vi "ExDisplayMultiple.vi"() -> ()   [LabVIEW 2010]
uses:
  GlobalCurrentFrame.vi
  GlobalFileInfo.vi
  GlobalLastFrame.vi
panel:
  out "Last Frame Number":u32
  in  "Stop 2":bool
  in  "Stop":bool
  out "Current Frame Number":u32
  in  "Go To End":bool
  in  "Go to begining":bool
  in  "Prev Frame":bool
  in  "Next Frame":bool
  in  "Full File Name":path
  out "error out":errorcluster
  in  "error in (no error)":errorcluster
  in  "SITKFULLDISPLAYLib.SITKFullDisplay":refnum<k7>(container)
  # "Browse match pattern is set to *.tif.  Modify this if different file type is needed."
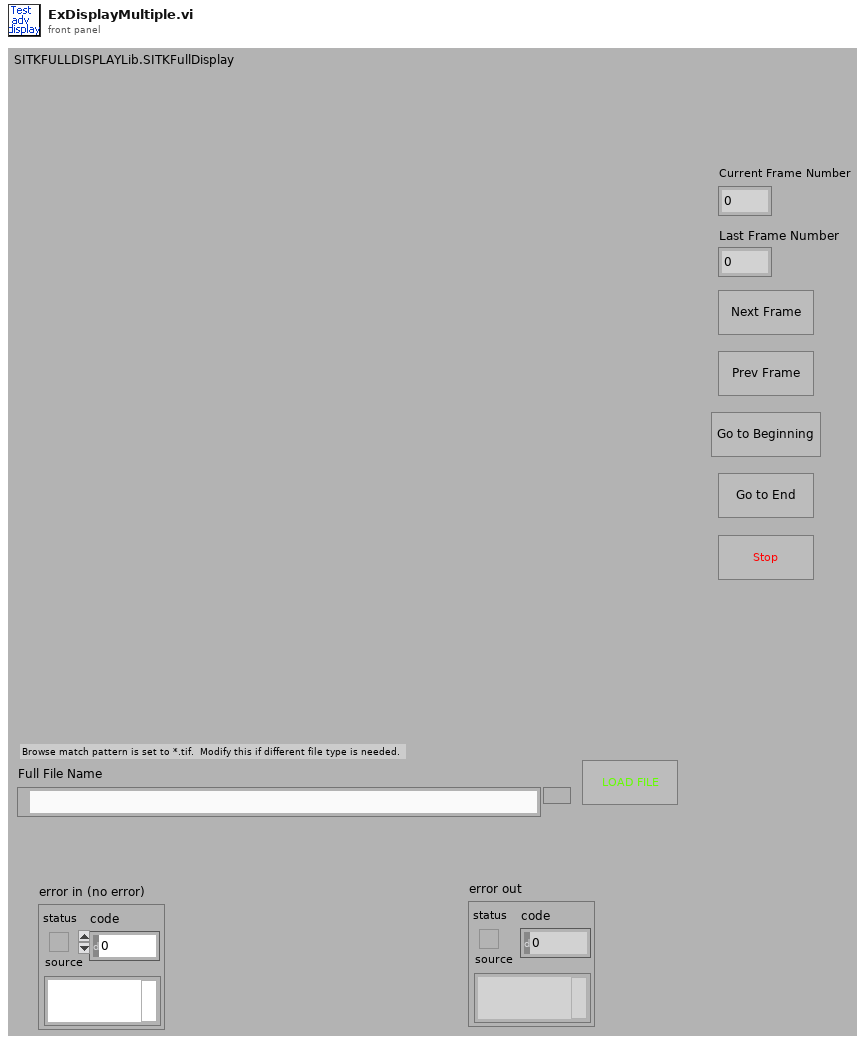
[diagram p1: front panel]
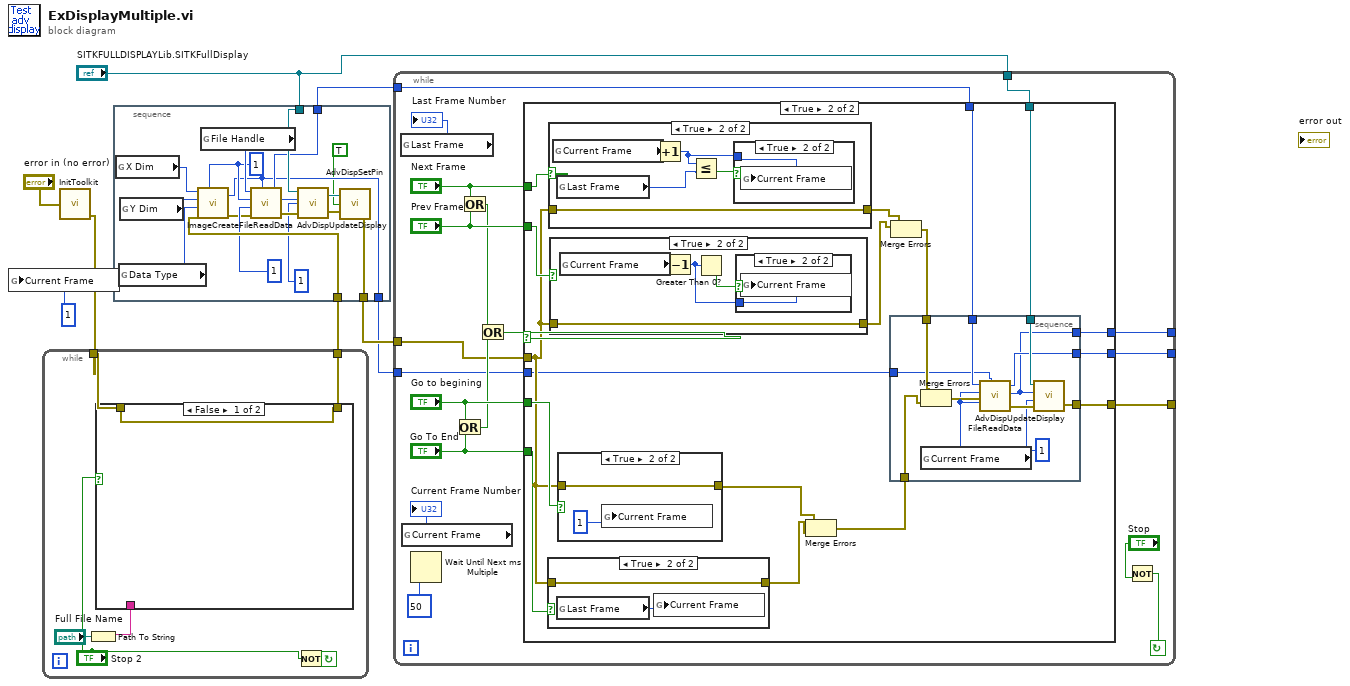
[diagram p0: block diagram]
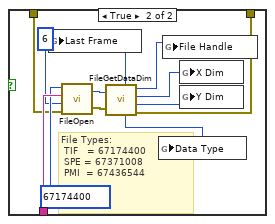
[diagram p2: hidden frame]
diagram:
  n1 = global write "GlobalCurrentFrame.vi" "Current Frame"(1) -> ()
  n2 = call <userlib>:"InitToolkit.vi"("error in"="error in (no error)") -> ("error out"=w4:errorcluster)
  n3 = while {
    tunnel: w4 -> [w12]
    tunnel: [w9] -> w3
    stop <- w10 continue-if-true
    n4 = Path To String(path="Full File Name") -> (string=w13:string)
    n5 = case shown="False" "Stop 2" {
      tunnel: w13 -> [_ w27]
      tunnel: w12 -> [w15 w21]
      tunnel: [w15 w16] -> w9
      frame False {
      }
      frame True {
        # "File Types:\n TIF   = 67174400\n SPE = 67371008\n PMI  = 67436544"
        n6 = call <userlib>:"FileOpen.vi"("error in"=w21, "File Operations"=6, "FileName"=w27, "File Type"=67174400) -> ("error out"=w26:errorcluster, "File Handle"=w25:u32)
        n7 = call <userlib>:"FileGetDataDim.vi"("File Handle"=w25, "error in"=w26) -> ("Number of Frames"=w23:u32, "Data Type"=w17:u32, "File Handle"=w20:u32, "X dim"=w19:u32, "Y dim"=w18:u32, "error out"=w16:errorcluster)
        n8 = global write "GlobalLastFrame.vi" "Last Frame"(w23) -> ()
        n9 = global write "GlobalFileInfo.vi" "Data Type"(w17) -> ()
        n10 = global write "GlobalFileInfo.vi" "File Handle"(w20) -> ()
        n11 = global write "GlobalFileInfo.vi" "X Dim"(w19) -> ()
        n12 = global write "GlobalFileInfo.vi" "Y Dim"(w18) -> ()
      }
    }
    n13 = Not(x="Stop 2") -> (.not. x?=w10:bool)
  }
  n14 = stacked-sequence {
    tunnel: [w30] -> w6
    tunnel: "SITKFULLDISPLAYLib.SITKFullDisplay" -> [w44]
    tunnel: w3 -> [w43]
    tunnel: [w37] -> w2
    tunnel: [w29] -> w1
    frame #0 {
      w34 = 1
      n15 = global read "GlobalFileInfo.vi" "X Dim"() -> (w40:u32)
      n16 = global read "GlobalFileInfo.vi" "Data Type"() -> (w42:u32)
      n17 = global read "GlobalFileInfo.vi" "Y Dim"() -> (w41:u32)
      n18 = call <userlib>:"ImageCreate.vi"("X dimension"=w40, "Y dimension"=w41, "Data Type"=w42, "error in"=w43, "Number Of Frames"=w34) -> ("Image Handle"=w29:u32, "error out"=w33:errorcluster)
      n19 = global read "GlobalFileInfo.vi" "File Handle"() -> (w38:u32)
      n20 = call <userlib>:"FileReadData.vi"("File Handle"=w38, "Start Frame"=w34, "End Frame"=1, "error in"=w33, "Image Handle"=w29) -> ("File Handle"=w37:u32, "Image Handle"=w36:u32, "error out"=w45:errorcluster)
      n21 = call <userlib>:"AdvDispUpdateDisplay.vi"("error in (no error)"=w45, "Frame Number To Display"=1, "Image Handle"=w36, "SITKFULLDISPLAYLib.SITKFullDisplay"=w44) -> ("error out"=w32:errorcluster, "SITKFULLDISPLAYLib.SITKFullDisplay"=w31:refnum<k7>)
      n22 = call <userlib>:"AdvDispSetPin.vi"("SITKFULLDISPLAYLib.SITKFullDisplay"=w31, "Pin Enable"=TRUE, "error in (no error)"=w32) -> ("error out"=w30:errorcluster)  [unwired: 3 out]
    }
  }
  n23 = while {
    tunnel: w2 -> [w55]
    tunnel: w6 -> [w54]
    tunnel: w1 -> [w53]
    tunnel: "SITKFULLDISPLAYLib.SITKFullDisplay" -> [w52]
    tunnel: [w49] -> _
    tunnel: [w48] -> _
    tunnel: [w47] -> _
    stop <- w50 continue-if-true
    n24 = global read "GlobalLastFrame.vi" "Last Frame"() -> (→"Last Frame Number":u32)
    n25 = global read "GlobalCurrentFrame.vi" "Current Frame"() -> (→"Current Frame Number":u32)
    n26 = Wait Until Next ms Multiple(millisecond multiple=50) -> ()  [unwired: 1 out]
    n27 = Or(x="Go to begining", y="Go To End") -> (x .or. y?=w58:bool)
    n28 = Or(x="Next Frame", y="Prev Frame") -> (x .or. y?=w57:bool)
    n29 = Or(x=w57, y=w58) -> (x .or. y?=w56:bool)
    n30 = case shown="True" w56 {
      tunnel: "Go To End" -> [_ w81]
      tunnel: "Go to begining" -> [_ w82]
      tunnel: "Prev Frame" -> [_ w83]
      tunnel: "Next Frame" -> [_ w84]
      tunnel: w55 -> [w66 w80]
      tunnel: w54 -> [w67 w79]
      tunnel: w53 -> [w65 w72]
      tunnel: w52 -> [_ w71]
      tunnel: [w67 w70] -> w49
      tunnel: [w66 w69] -> w48
      tunnel: [w65 w68] -> w47
      frame False {
      }
      frame True {
        n31 = case shown="True" w81 {
          tunnel: w79 -> [w97 w98]
          tunnel: [w97 w98] -> w75
          frame False {
          }
          frame True {
            n32 = global read "GlobalLastFrame.vi" "Last Frame"() -> (w99:u32)
            n33 = global write "GlobalCurrentFrame.vi" "Current Frame"(w99) -> ()
          }
        }
        n34 = case shown="True" w84 {
          tunnel: w79 -> [w109 w110]
          tunnel: [w109 w110] -> w78
          frame False {
          }
          frame True {
            n35 = global read "GlobalCurrentFrame.vi" "Current Frame"() -> (w114:u32)
            n36 = global read "GlobalLastFrame.vi" "Last Frame"() -> (w113:u32)
            n37 = Increment(x=w114) -> (x+1=w111:u32)
            n38 = Less Or Equal?(x=w111, y=w113) -> (x <= y?=w112:bool)
            n39 = case shown="True" w112 {
              tunnel: w111 -> [_ w115]
              frame False {
              }
              frame True {
                n40 = global write "GlobalCurrentFrame.vi" "Current Frame"(w115) -> ()
              }
            }
          }
        }
        n41 = case shown="True" w83 {
          tunnel: w79 -> [w103 w104]
          tunnel: [w103 w104] -> w77
          frame False {
          }
          frame True {
            n42 = global read "GlobalCurrentFrame.vi" "Current Frame"() -> (w107:u32)
            n43 = Decrement(x=w107) -> (x-1=w105:u32)
            n44 = Greater Than 0?(x=w105) -> (x > 0?=w106:bool)
            n45 = case shown="True" w106 {
              tunnel: w105 -> [_ w108]
              frame False {
              }
              frame True {
                n46 = global write "GlobalCurrentFrame.vi" "Current Frame"(w108) -> ()
              }
            }
          }
        }
        n47 = case shown="True" w82 {
          tunnel: w79 -> [w100 w101]
          tunnel: [w100 w101] -> w76
          frame False {
          }
          frame True {
            n48 = global write "GlobalCurrentFrame.vi" "Current Frame"(1) -> ()
          }
        }
        n49 = Merge Errors(w76, w75) -> (w73:errorcluster)
        n50 = Merge Errors(w78, w77) -> (w74:errorcluster)
        n51 = stacked-sequence {
          tunnel: w80 -> [w96]
          tunnel: w74 -> [w95]
          tunnel: w73 -> [w94]
          tunnel: w72 -> [w92]
          tunnel: w71 -> [w90]
          tunnel: [w87] -> w70
          tunnel: [w86] -> w69
          tunnel: [w85] -> w68
          frame #0 {
            n52 = Merge Errors(w95, w94) -> (w93:errorcluster)
            n53 = global read "GlobalCurrentFrame.vi" "Current Frame"() -> (w89:u32)
            n54 = call <userlib>:"FileReadData.vi"("File Handle"=w96, "Start Frame"=w89, "End Frame"=w89, "error in"=w93, "Image Handle"=w92) -> ("File Handle"=w86:u32, "Image Handle"=w85:u32, "error out"=w91:errorcluster)
            n55 = call <userlib>:"AdvDispUpdateDisplay.vi"("error in (no error)"=w91, "Frame Number To Display"=1, "Image Handle"=w85, "SITKFULLDISPLAYLib.SITKFullDisplay"=w90) -> ("error out"=w87:errorcluster)  [unwired: 1 out]
          }
        }
      }
    }
    n56 = Not(x="Stop") -> (.not. x?=w50:bool)
  }
